vi "test_settime.vi"() -> ()   [LabVIEW 2017]
uses:
  <vilib>/nisyscfg/nisyscfg.lvlib
panel:
  out "Detailed Result":string
  out "error out":errorcluster
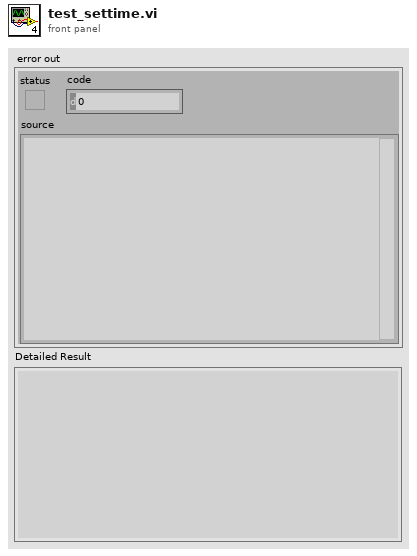
[diagram p1: front panel]
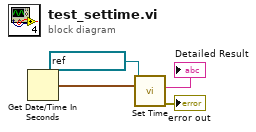
[diagram p0: block diagram]
diagram:
  n1 = Get Date/Time In Seconds() -> (seconds since 1Jan1904=w3:timestamp)
  n2 = call <vilib>:"Set Time.vi"("Time"=w3, "Session in (localhost)"=refnum<k21> "localhost") -> ("error out"=→"error out":errorcluster, "Detailed Result"=→"Detailed Result":string)  [unwired: 6 in, 2 out]
